vi "실습 5-2.vi"() -> ()   [LabVIEW 2014]
panel:
  out "추가된 배열":string[](array[string])
  out "에러 출력":errorcluster
  in  "머신 이름(\"\":  로컬 참조 열기)":string
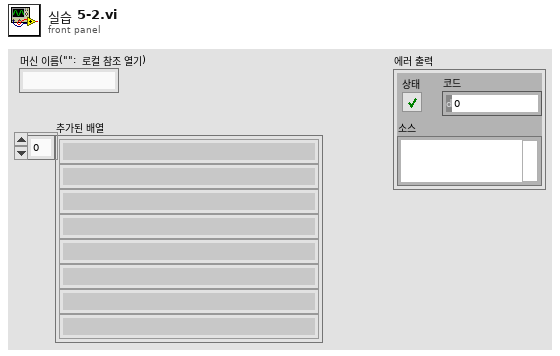
[diagram p1: front panel]
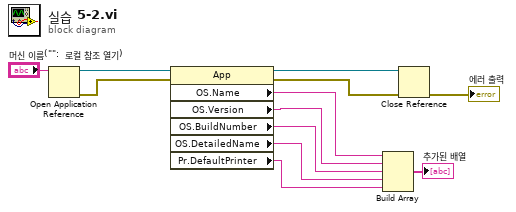
[diagram p0: block diagram]
diagram:
  n1 = Open Application Reference(11:"머신 이름(\"\":  로컬 참조 열기)") -> (0:w11:errorcluster, 3:w1:refnum<vi>)  [unwired: 3 in]
  n2 = property class="App"(reference=w1, error in=w11) -> (reference out=w10:refnum<vi>, error out=w9:errorcluster, "OS.Name"=w7:string, "OS.Version"=w6:string, "OS.BuildNumber"=w5:string, "OS.DetailedName"=w4:string, "Pr.DefaultPrinter"=w3:string)
  n3 = Build Array(w7, w6, w5, w4, w3) -> (→"추가된 배열":string[])
  n4 = Close Reference(reference=w10, error in (no error)=w9) -> (error out=→"에러 출력":errorcluster)
